vi "setUp.vi"(8 "error in (no error)":errorcluster, 11 "reference in":refnum<class "FPGA Addon DMA Waveform Status Channel System Tests.lvclass">) -> (0 "error out":errorcluster, 3 "reference out":refnum<class "FPGA Addon DMA Waveform Status Channel System Tests.lvclass">)   [LabVIEW 2018, in "FPGA Addon DMA Waveform Status Channel System Tests.lvclass"]
doc: "setUp runs prior to the test method during test execution. Use this method to initialize any object data required by your tests."
uses:
  FPGA Addon DMA Waveform Status Channel System Tests.lvclass
  C:/Users/nitest/Desktop/NI VS FPGA Addon CD Fork/Source/Tests/FPGA Addon Test Class/FPGA Addon Test Class.lvclass
  C:/Program Files (x86)/National Instruments/LabVIEW 2018/vi.lib/addons/_JKI Toolkits/VI Tester/TestCase.llb/TestCase.lvclass
  FPGA Addon Test Class/FPGA Addon Test Class.lvclass/FPGA Addon Test Class.ctl
  <vilib>/addons/_JKI Toolkits/VI Tester/TestCase.llb/TestCase.lvclass
  FPGA Addon Test Class/FPGA Addon Test Class.lvclass
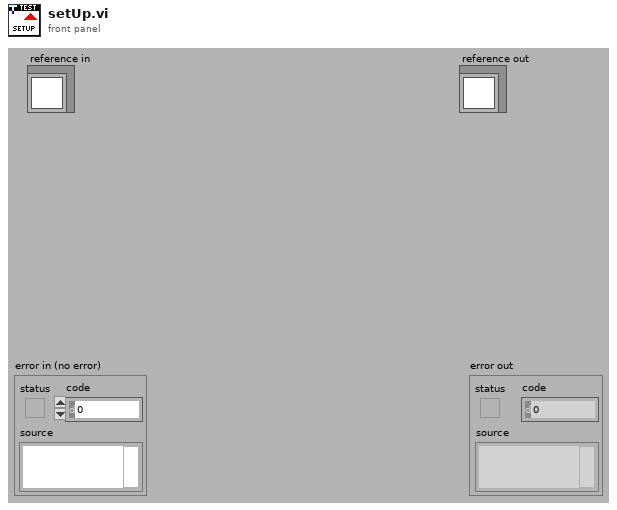
[diagram p1: front panel]
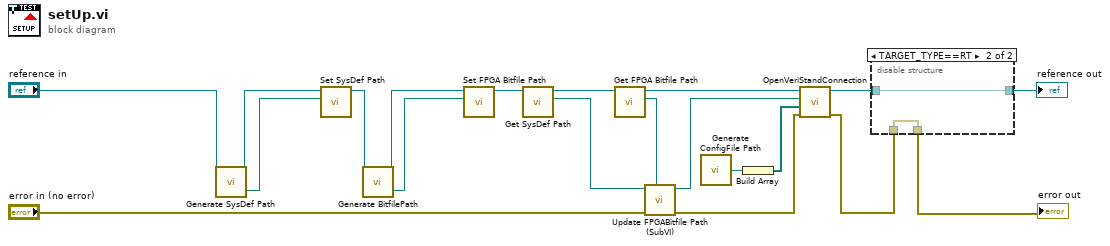
[diagram p0: block diagram]
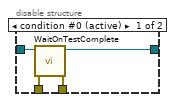
[diagram p2: hidden frame]
diagram:
  n1 = call "Generate SysDef Path.vi"("reference in"="reference in") -> ("SysDef path"=w14:path, "reference out"=w10:refnum<class "FPGA Addon DMA Waveform Status Channel System Tests.lvclass">)  [unwired: 1 in]
  n2 = call "Set SysDef Path.vi"("SysDef Path"=w14, "Scalar Channels Testing in"=w10) -> ("Scalar Channels Testing out"=w9:refnum<class "FPGA Addon DMA Waveform Status Channel System Tests.lvclass">)  [unwired: 9 in]
  n3 = call "Generate BitfilePath.vi"("reference in"=w9) -> ("Bitfile path"=w13:path, "reference out"=w8:refnum<class "FPGA Addon DMA Waveform Status Channel System Tests.lvclass">)  [unwired: 1 in]
  n4 = call "Set FPGA Bitfile Path.vi"("FPGA Bitfile Path"=w13, "Scalar Channels Testing in"=w8) -> ("Scalar Channels Testing out"=w18:refnum<class "FPGA Addon DMA Waveform Status Channel System Tests.lvclass">)  [unwired: 9 in]
  n5 = call "Get SysDef Path.vi"("Scalar Channels Testing in"=w18) -> ("SysDef Path"=w15:path, "Scalar Channels Testing out"=w17:refnum<class "FPGA Addon DMA Waveform Status Channel System Tests.lvclass">)  [unwired: 9 in]
  n6 = call "Get FPGA Bitfile Path.vi"("Scalar Channels Testing in"=w17) -> ("FPGA Bitfile Path"=w16:path, "Scalar Channels Testing out"=w7:refnum<class "FPGA Addon DMA Waveform Status Channel System Tests.lvclass">)  [unwired: 9 in]
  n7 = call "Update FPGABitfile Path (SubVI).vi"("Bitfile Path"=w16, "error in (no error)"="error in (no error)", "System Definition path in"=w15) -> ("error out"=w5:errorcluster, "System Definition path out"=w3:path)  [unwired: 7 in]
  n8 = call "Generate ConfigFile Path.vi"() -> ("ConfigFile path"=w2:path)
  n9 = Build Array(w2) -> (w1:path[])
  n10 = call-dynamic "OpenVeriStandConnection.vi"("error in (no error)"=w5, "overrides files"=w1, "System Definition File"=w3, "VeriStand Test Case in"=w7) -> ("error out"=w4:errorcluster, "VeriStand Test Case out"=w6:refnum<class "FPGA Addon DMA Waveform Status Channel System Tests.lvclass">)  [unwired: 5 in, 1 out]
  n11 = disable-structure shown="TARGET_TYPE==RT" {
    disable-tunnel: w4 -> [w24 w25]
    disable-tunnel: [w23 w25] -> w20
    disable-tunnel: [w22 w26] -> w19
    disable-tunnel: w6 -> [w21 w26]
    frame condition #0 (active) {
      n12 = call <vilib>:"WaitOnTestComplete.vi"("error in (no error)"=w24, "TestCase in"=w21) -> ("error out"=w23:errorcluster, "TestCase out"=w22:refnum<class "FPGA Addon DMA Waveform Status Channel System Tests.lvclass">)  [unwired: 8 in]
    }
    frame condition #1 {
    }
  }
  "error out" <- w20
  "reference out" <- w19
